vi "WPI_SerialPortOpen.vi"(0 "Baud Rate":u32=9600, 1 "Timeout Value (ms)":u32=5000, 2 "Termination Char (0xA = '\\n' = LF)":u8=10 format="%.0x", 3 "Enable Termination Char? (T)":bool=TRUE, 5 "Data Bits":u16=8, 7 "Parity":u16(ring) items=["None", "Odd", "Even", "Mark", "Space"], 9 "Stop Bits":u16(ring)=10 items=["1.0"=10, "1.5"=15, "2.0"=20], 11 "error in (no error)":errorcluster, 12 "Flow Control":u16(ring) items=["None", "XON/XOFF", "RTS/CTS", "XON/XOFF & RTS/CTS", "DTR/DSR", "XON/XOFF & DTR/DSR"], 13 "Serial Port":T1) -> (4 "SerialPortRef":T2, 15 "error out":errorcluster)   [LabVIEW 2017]
doc: "Opens a reference to the serial port. You must open a reference before using any other VIs on this palette.\n\nThis software is licensed. Open the labview\\readme\\WPI Robotics Library Open Source License.txt file for more information."
uses:
  <vilib>/Rock Robotics/WPI/SerialPort/WPI_SerialPortRef.ctl
  <vilib>/Rock Robotics/WPI/SerialPort/WPI_SerialPort.ctl
  <vilib>/Rock Robotics/SystemInterfaces/NetworkCommunication/NetComm_UsageReport_ResourceType.ctl
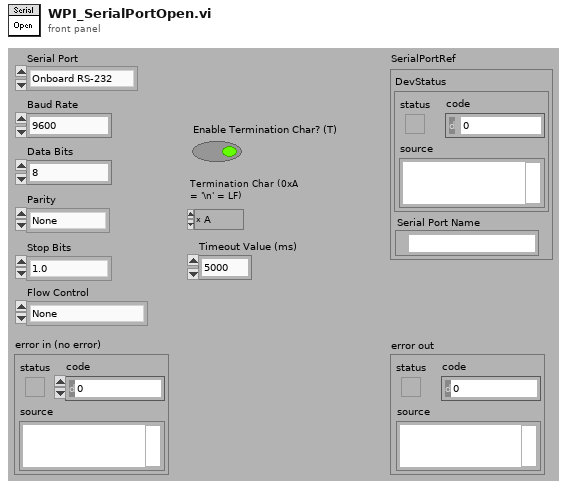
[diagram p1: front panel]
types:
  T1 = typedef "WPI_SerialPort.ctl" = enum16{"Onboard RS-232", "MXP TTL", "USB 1", "USB 2"}
  T2 = typedef "WPI_SerialPortRef.ctl" = cluster{"DevStatus":errorcluster, "Serial Port Name":refnum<visa-resource-name>}
  T3 = typedef "NetComm_UsageReport_ResourceType.ctl" = enum8{"Controller", "Module", "Language", "CANPlugin", "Accelerometer", "ADXL345", "AnalogChannel", "AnalogTrigger", "AnalogTriggerOutput", "CANJaguar", "Compressor", "Counter", "Dashboard", "DigitalInput", "DigitalOutput", "DriverStationCIO", "DriverStationEIO", "DriverStationLCD", "Encoder", "GearTooth", "Gyro", "I2C", "Framework", "Jaguar", "Joystick", "Kinect", "KinectStick", "PIDController", "Preferences", "PWM", "Relay", "RobotDrive", "SerialPort", "Servo", "Solenoid", "SPI", "Task", "Ultrasonic", "Victor", "Button", "Command", "AxisCamera", "PCVideoServer", "SmartDashboard", "Talon", "HiTechnicColorSensor", "HiTechnicAccel", "HiTechnicCompass", "SRF08", "AnalogOutput", "Victor SP", "Talon SRX", "CAN Talon SRX", "ADXL362 Accel", "ADXRS450 Gyro", "Rev SPARK", "Mindsensors SD540", "Digital Filter", "ADIS16448", "PDP", "PCM", "PigeonIMU", "Nidec Brushless", "CTRE CANifier", "CTRE Future 0", "CTRE Future 1", "CTRE Future 2", "CTRE Future 3", "CTRE Future 4", "CTRE Future 5", "CTRE Future 6"}
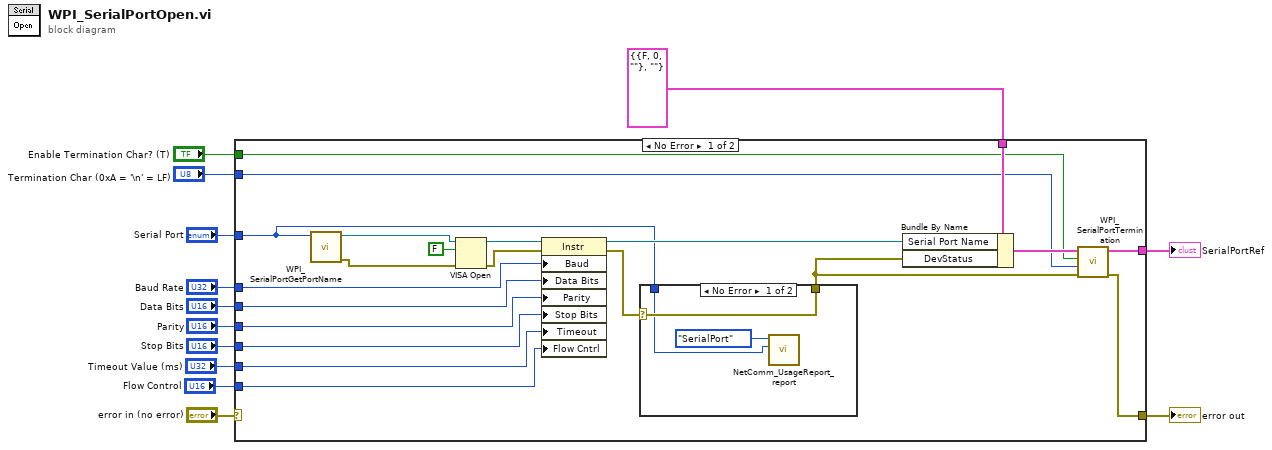
[diagram p0: block diagram]
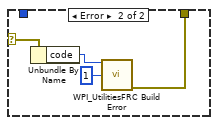
[diagram p2: hidden frame]
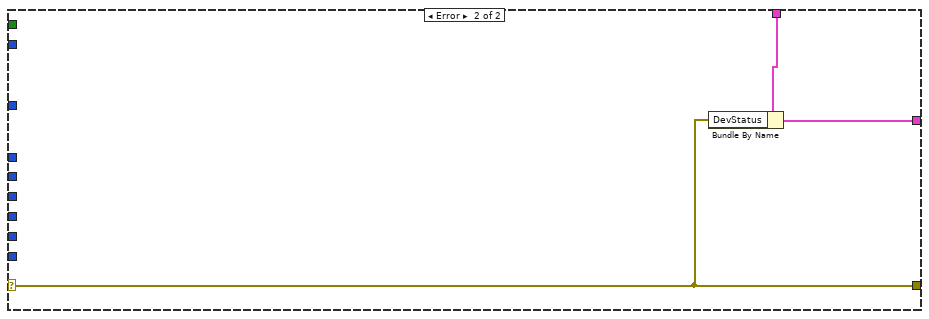
[diagram p3: hidden frame]
diagram:
  n1 = case shown="No Error" "error in (no error)" {
    selector: "error in (no error)" -> [_ w43]
    tunnel: "Baud Rate" -> [w32 _]
    tunnel: "Parity" -> [w31 _]
    tunnel: "Data Bits" -> [w30 _]
    tunnel: [w24 w44] -> w10
    tunnel: "Stop Bits" -> [w20 _]
    tunnel: [w25 w43] -> w7
    tunnel: T2 {"DevStatus"={"status"=FALSE, "code"=0, "source"=""}, "Serial Port Name"=""} ("SerialPortRef") -> [w28 w42]
    tunnel: "Enable Termination Char? (T)" -> [w22 _]
    tunnel: "Termination Char (0xA = '\\n' = LF)" -> [w23 _]
    tunnel: "Timeout Value (ms)" -> [w21 _]
    tunnel: "Flow Control" -> [w19 _]
    tunnel: "Serial Port" -> [w14 _]
    frame No Error {
      n2 = call <vilib>:"WPI_SerialPortGetPortName.vi"("Serial Port"=w14) -> ("error out"=w15:errorcluster, "VISA Refnum out"=w16:refnum<visa-resource-name>)  [unwired: 9 in]
      n3 = VISA Open(duplicate session (F)=FALSE, error in (no error)=w15, VISA resource name=w16) -> (VISA resource name=w34:refnum<visa-resource-name>, error out=w33:errorcluster)  [unwired: 2 out]
      n4 = property class="Instr"(reference=w34, error in=w33, "Baud"=w32, "Data Bits"=w30, "Parity"=w31, "Stop Bits"=w20, "Timeout"=w21, "Flow Cntrl"=w19) -> (reference out=w29:refnum<visa-resource-name>, error out=w18:errorcluster)
      n5 = case shown="No Error" w18 {
        selector: w18 -> [w37 w39]
        tunnel: [w37 w38] -> w17
        tunnel: w14 -> [w35 _]
        frame No Error {
          n6 = call <vilib>:"NetComm_UsageReport_report.vi"("Instance Number"=w35, "Resource Type"=NetComm_UsageReport_ResourceType."SerialPort") -> ()  [unwired: 10 in]
        }
        frame Error {
          n7 = Unbundle By Name(w39) -> ("code"=w41:i32)
          n8 = call <vilib>:"WPI_UtilitiesFRC Build Error.vi"("error code"=w41, "chain levels to remove (1)"=1) -> ("error out"=w38:errorcluster)  [unwired: 3 in, 10 out]
        }
      }
      n9 = Bundle By Name(cluster=w28, "Serial Port Name"=w29, "DevStatus"=w17) -> (w26:T2)
      n10 = call <vilib>:"WPI_SerialPortTermination.vi"("error in (no error)"=w17, "Termination Char (0xA = '\\n' = LF)"=w23, "Enable? (T)"=w22, "SerialPortRef"=w26) -> ("error out"=w25:errorcluster, "SerialPortRef"=w24:T2)  [unwired: 6 out]
    }
    frame Error {
      n11 = Bundle By Name(cluster=w42, "DevStatus"=w43) -> (w44:T2)
    }
  }
  "error out" <- w7
  "SerialPortRef" <- w10
